vi "Packages List Path--constant.vi"(8 "error in (no error)":errorcluster, 11 "LabVIEW Web Service":refnum<class "Web Service.lvclass">) -> (0 "error out":errorcluster, 2 "Packages index path":path, 3 "LabVIEW Web Service out":refnum<class "Web Service.lvclass">)   [LabVIEW 2020, in "WSsupport.lvlib"]
uses:
  WSsupport.lvlib
  <vilib>/wsapi/Web Service.lvclass
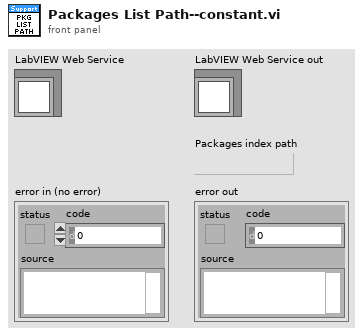
[diagram p1: front panel]
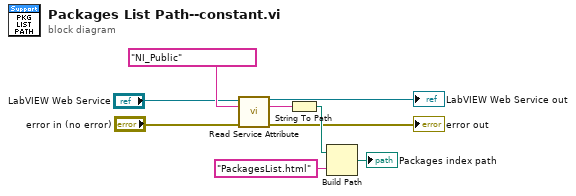
[diagram p0: block diagram]
diagram:
  n1 = call <vilib>:"Read Service Attribute.vi"("LabVIEW Web Service"="LabVIEW Web Service", "attribute name"="NI_Public", "error in (no error)"="error in (no error)") -> ("LabVIEW Web Service out"=→"LabVIEW Web Service out":refnum<class "Web Service.lvclass">, "value"=w8:string, "error out"=→"error out":errorcluster)  [unwired: 10 in]
  n2 = String To Path(string=w8) -> (path=w7:path)
  n3 = Build Path(base path=w7, name or relative path="PackagesList.html") -> (appended path=→"Packages index path":path)
